vi "editScriptEvent.vi"(8 "error in (no error)":errorcluster, 11 "ScriptEditorV2 in":refnum<class "ScriptEditorV2.lvclass">) -> (0 "error out":errorcluster, 3 "ScriptEditorV2 out":refnum<class "ScriptEditorV2.lvclass">)   [LabVIEW 2009, in "Views.lvlib" / "ScriptEditor.lvlib" / "ScriptEditorV2.lvclass"]
uses:
  ScriptEditorV2.lvclass
  EventEditor/ActionEditor/ActionEditor.lvclass
  ScriptEditorV2.lvclass/ScriptEditorV2.ctl
  Tools/Scripting/ScriptingEvent/ScriptEventList/ScriptEventList.lvclass
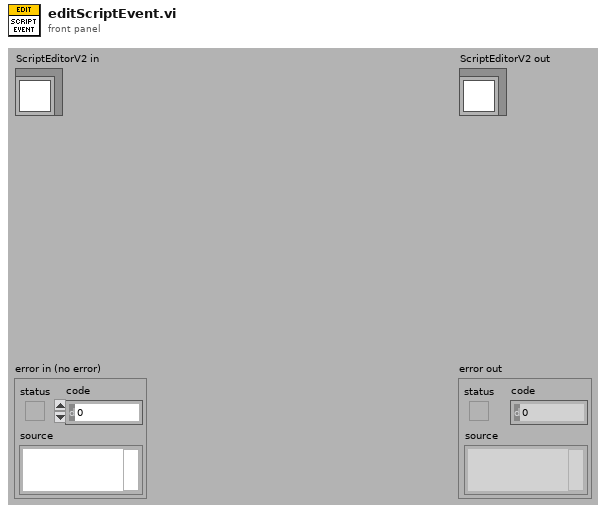
[diagram p1: front panel]
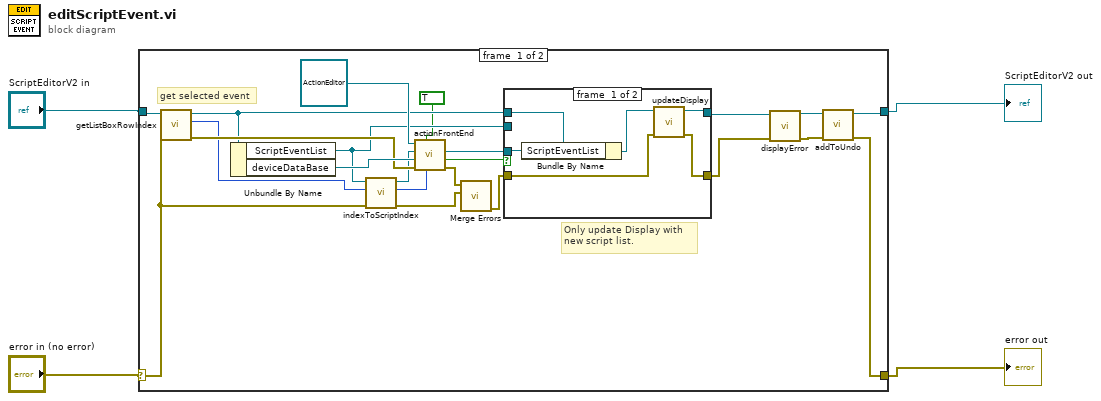
[diagram p0: block diagram]
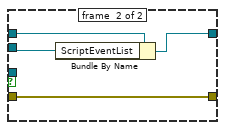
[diagram p2: hidden frame]
diagram:
  n1 = case shown="No Error" "error in (no error)" {
    selector: "error in (no error)" -> [w14 w38]
    tunnel: [w5 w38] -> w1
    tunnel: [w7 w37] -> w2
    tunnel: "ScriptEditorV2 in" -> [w26 w37]
    frame #0 {
      # "get selected event"
      # "Only update Display with\nnew script list."
      n2 = call "getListBoxRowIndex.vi"("error in (no error)"=w14, "ScriptEditorV2 in"=w26) -> ("error out"=w24:errorcluster, "rowIndex"=w18:i32, "ScriptEditorV2 out"=w10:refnum<class "ScriptEditorV2.lvclass">)  [unwired: 7 in]
      n3 = Unbundle By Name(w10) -> ("ScriptEventList"=w16:refnum<class "ScriptEventList.lvclass">, "deviceDataBase"=w25:refnum<class "deviceDataBase.lvclass">)
      n4 = call "indexToScriptIndex.vi"("error in (no error)"=w14, "sequencedIndex"=w18, "ScriptEventList in"=w16) -> ("error out"=w11:errorcluster, "indexScriptEvent"=w17:i32, "ScriptEventList out"=w15:refnum<class "ScriptEventList.lvclass">)  [unwired: 6 in]
      n5 = call-dynamic "actionFrontEnd.vi"("index"=w17, "editing"=TRUE, "error in (no error)"=w24, "deviceDataBase"=w25, "ScriptEventList"=w15, "ActionEditor in"=refnum<class "ActionEditor.lvclass"> refnum ("Views.lvlib:SciptEditor.lvlib:ActionEditor.lvclass")) -> ("error out"=w13:errorcluster, "canceled"=w22:bool, "ScriptEventList out"=w21:refnum<class "ScriptEventList.lvclass">)  [unwired: 2 in, 1 out]
      n6 = call <vilib>:"Merge Errors.vi"("error in 2 (no error)"=w11, "error in 1 (no error)"=w13) -> ("error out"=w12:errorcluster)  [unwired: 5 in]
      n7 = case shown="False" w22 {
        tunnel: w10 -> [w31 w35]
        tunnel: [w29 w34] -> w20
        tunnel: w12 -> [w28 w33]
        tunnel: w21 -> [w32 _]
        tunnel: w16 -> [_ w36]
        tunnel: [w27 w33] -> w19
        frame #0 {
          n8 = Bundle By Name(cluster=w31, "ScriptEventList"=w32) -> (w30:refnum<class "ScriptEditorV2.lvclass">)
          n9 = call "updateDisplay.vi"("error in (no error)"=w28, "ScriptEditorV2 in"=w30) -> ("error out"=w27:errorcluster, "ScriptEditorV2 out"=w29:refnum<class "ScriptEditorV2.lvclass">)  [unwired: 8 in]
        }
        frame #1 {
          n10 = Bundle By Name(cluster=w35, "ScriptEventList"=w36) -> (w34:refnum<class "ScriptEditorV2.lvclass">)
        }
      }
      n11 = call "displayError.vi"("error in (no error)"=w19, "ScriptEditorV2 in"=w20) -> ("error out"=w6:errorcluster, "ScriptEditorV2 out"=w8:refnum<class "ScriptEditorV2.lvclass">)  [unwired: 8 in]
      n12 = call "addToUndo.vi"("error in (no error)"=w6, "ScriptEditorV2 in"=w8) -> ("error out"=w5:errorcluster, "ScriptEditorV2 out"=w7:refnum<class "ScriptEditorV2.lvclass">)  [unwired: 8 in]
    }
    frame #1 {
    }
  }
  "error out" <- w1
  "ScriptEditorV2 out" <- w2
